vi "Configure Scan Engine and EtherCAT Custom Device.vi"() -> ()   [LabVIEW 2019]
uses:
  <vilib>/addons/VeriStand Custom Device Scripting APIs/Scan Engine/Modules/Mode Classes/Controls/digital channel settings.ctl
  <vilib>/addons/VeriStand Custom Device Scripting APIs/Scan Engine/Modules/Mode Classes/Controls/counter driven output channel settings.ctl
  <vilib>/addons/VeriStand Custom Device Scripting APIs/Scan Engine/Modules/Channel Classes/Counter Driven Output Channel/Counter Driven State.ctl
  <vilib>/addons/VeriStand Custom Device Scripting APIs/Scan Engine/Scan Engine Dependencies.llb/Local Chassis Settings.ctl
  <vilib>/addons/VeriStand Custom Device Scripting APIs/Scan Engine/Modules/Mode Classes/Counter Driven Output Mode/Drive from Slot.ctl
  <vilib>/addons/VeriStand Custom Device Scripting APIs/Scan Engine/Scan Engine Dependencies.llb/Main Settings.ctl
  NationalInstruments.VeriStand.SystemDefinitionAPI
  <vilib>/addons/VeriStand Custom Device Scripting APIs/Scan Engine/Modules/NI 9474/NI 9474.lvclass
  C:/Program Files (x86)/National Instruments/LabVIEW 2019/vi.lib/addons/VeriStand Custom Device Scripting APIs/Scan Engine/Modules/Module/Module.lvclass
  <vilib>/addons/VeriStand Custom Device Scripting APIs/Scan Engine/Modules/NI 9475/NI 9475.lvclass
  <vilib>/addons/VeriStand Custom Device Scripting APIs/Scan Engine/Modules/NI 9474/Create NI 9474 - Digital Output.vi
  <vilib>/addons/VeriStand Custom Device Scripting APIs/Scan Engine/Modules/NI 9475/Create NI 9475 - Counter Driven Output.vi
  SubVIs/Scan Engine Example Support.lvlib
  <vilib>/addons/VeriStand Custom Device Scripting APIs/Scan Engine/Scan Engine Scripting.lvlib
  <vilib>/addons/VeriStand Custom Device Scripting APIs/Scan Engine/Modules/Channel Classes/Counter Driven Output Channel/Counter Driven Output Channel.lvclass
  <vilib>/addons/VeriStand Custom Device Scripting APIs/Scan Engine/Scan Engine Dependencies.llb/Scan Engine Custom Device.lvlib
  <vilib>/addons/VeriStand Custom Device Scripting APIs/Scan Engine/Modules/Mode Classes/Counter Driven Output Mode/Counter Driven Output Mode.lvclass
panel:
  in  "Output System Definition File":path=path "System Definition Files/Scripted Scan Engine.nivssdf"
  in  "Input System Definition File":path=path "System Definition Files/Base.nivssdf"
  # "Overview: Demonstrates using the Scan Engine and EtherCAT scripting API to configure the custom device. \n\nInstructions:\n1. Browse to a system definition file to be used as the Input System Definition File that you would like to add a Scan Engine and EtherCAT custom device. This system defintion file should not already include a Scan Engine and EtherCAT custom device.\n2. Enter a path to save the system definition file as the Output System Definition File. \n3. Run the VI and verify its results in the VeriStand System Explorer."
  # "System Definition Files"
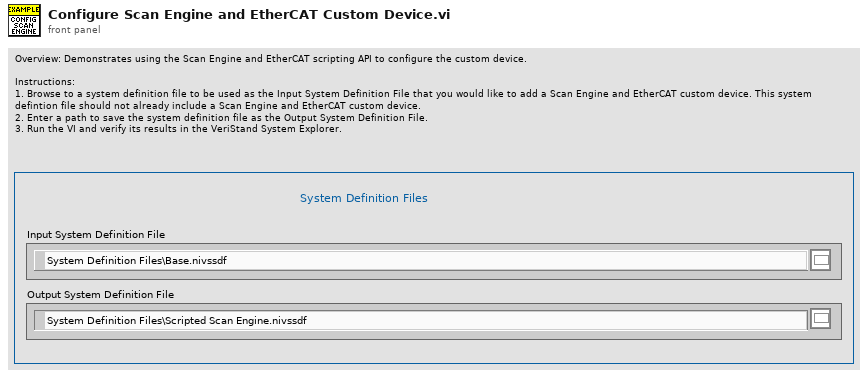
[diagram p1: front panel]
types:
  T1 = typedef "Scan Engine Custom Device.lvlib/Main Settings.ctl" = cluster{"sync to scan":bool, "scan engine decimation":u16, "delay after FPGA load (s)":u16}
  T2 = typedef "Scan Engine Scripting.lvlib/Counter Driven Output Mode.lvclass/Drive from Slot.ctl" = enum16{"Slot 1", "Slot 2", "Slot 3", "Slot 4", "Slot 5", "Slot 6", "Slot 7", "Slot 8"}
  T3 = typedef "Scan Engine Custom Device.lvlib/Local Chassis Settings.ctl" = cluster{"name":string, "number of slots":i32}
  T4 = typedef "Scan Engine Scripting.lvlib/counter driven output channel settings.ctl" = cluster{"name":string, "default value":bool, "counter driven state":T5}
  T5 = typedef "Scan Engine Scripting.lvlib/Counter Driven Output Channel.lvclass/Counter Driven State.ctl" = enum16{"Disabled", "Enabled"}
  T6 = typedef "Scan Engine Scripting.lvlib/digital channel settings.ctl" = cluster{"name":string, "default value":bool}
  T7 = typedef "Custom Device API.lvlib/Custom Device Item Ref.ctl" = u64
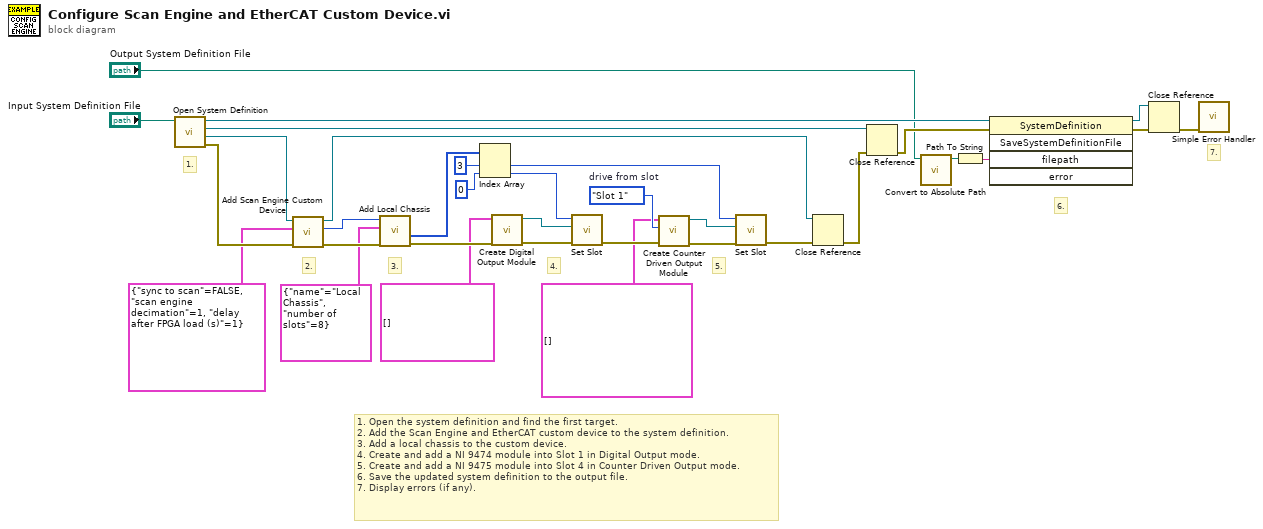
[diagram p0: block diagram]
diagram:
  w2 = Drive_from_Slot."Slot 1"  # drive from slot
  # "5."
  # "4."
  # "3."
  # "2."
  # "6."
  # "7."
  # "8."
  # "1."
  # "1. Open the system definition and find the first target.\n2. Add the Scan Engine and EtherCAT custom device to the system definition.\n3. Add a local chassis to the custom device.\n4. Create and add a NI 9474 module into Slot 1 in Digital Output mode. \n5. Create and add a NI 9475 module into Slot 4 in Counter Driven Output mode. \n6. Save the updated system definition to the output file.\n7. Display errors (if any)."
  n1 = call "Open System Definition.vi"("System Definition File"="Input System Definition File") -> ("error out"=w21:errorcluster, "Target Refnum"=w23:refnum<k24>, "Root Refnum"=w29:refnum<k24>, "System Definition Refnum"=w33:refnum<k24>)  [unwired: 7 in]
  n2 = call <vilib>:"Add Scan Engine Custom Device.vi"("error in"=w21, "settings"=T1 {"sync to scan"=FALSE, "scan engine decimation"=1, "delay after FPGA load (s)"=1}, "target in"=w23) -> ("error out"=w18:errorcluster, "scan engine custom device ref"=w19:T7, "target out"=w22:refnum<k24>)  [unwired: 6 in]
  n3 = call <vilib>:"Add Local Chassis.vi"("error in"=w18, "settings"=T3 {"name"="Local Chassis", "number of slots"=8}, "scan engine custom device ref in"=w19) -> ("error out"=w17:errorcluster, "slot refs"=w10:T7[])  [unwired: 4 in, 3 out]
  n4 = Index Array(array=w10, index #1=3 ("index"), index #2=0 ("index")) -> (element #1=w8:T7, element #2=w9:T7)
  n5 = call-poly <vilib>:"Create Digital Output Module.vi"("error in"=w17, "channel settings"=T6[] []) -> ("error out"=w16:errorcluster, "NI 9474 out"=w15:refnum<class "NI 9474.lvclass">)  [unwired: 8 in]
  n6 = call <vilib>:"Set Slot.vi"("error in"=w16, "module"=w15, "slot ref in"=w9) -> ("error out"=w14:errorcluster)  [unwired: 7 in, 1 out]
  n7 = call-poly <vilib>:"Create Counter Driven Output Module.vi"("error in"=w14, "drive from slot"=w2, "channel settings"=T4[] []) -> ("error out"=w13:errorcluster, "NI 9475 out"=w12:refnum<class "NI 9475.lvclass">)  [unwired: 7 in]
  n8 = call <vilib>:"Set Slot.vi"("error in"=w13, "module"=w12, "slot ref in"=w8) -> ("error out"=w11:errorcluster)  [unwired: 7 in, 1 out]
  n9 = Close Reference(reference=w22, error in (no error)=w11) -> (error out=w26:errorcluster)
  n10 = Close Reference(reference=w29, error in (no error)=w26) -> (error out=w28:errorcluster)
  n11 = call "Convert to Absolute Path.vi"("System Definition File"="Output System Definition File") -> ("Absolute Path"=w20:path)  [unwired: 10 in]
  n12 = Path To String(path=w20) -> (string=w32:string)
  n13 = invoke class="SystemDefinition" method="SaveSystemDefinitionFile"(reference=w33, error in=w28, "filepath"=w32) -> (reference out=w30:refnum<k24>, error out=w31:errorcluster)  [unwired: 2 in, 3 out]
  n14 = Close Reference(reference=w30, error in (no error)=w31) -> (error out=w25:errorcluster)
  n15 = call <vilib>:"Simple Error Handler.vi"("error in (no error)"=w25) -> ()  [unwired: 1 in, 8 out]
